vi "RIGOL_DS1202_continuous.vi"() -> ()   [LabVIEW 2021]
uses:
  <instrlib>/RIGOL DS1000 Series/Public/Data/Read (Single Waveform).vi
  <instrlib>/RIGOL DS1000 Series/RIGOL DS1000 Series.lvlib
panel:
  out "size(s)":i32
  in  "Channel (0: Channel 1)":u16(ring) items=["Channel 1", "Channel 2", "Channel 3", "Channel 4"]
  out "Waveform Data":waveform(dbl)(graph)={"t0"=timestamp(0 s since 1904-01-01), "dt"=2.0000000000000002e-07, "Y"=array[1202 elements]}
  in  "Stop":bool
  in  "Timeout (10000 ms)":u32=10000
  in  "VISA resource name":refnum<visa-resource-name>="USB0::0x1AB1::0x0517::DS1ZE244412916::INSTR"
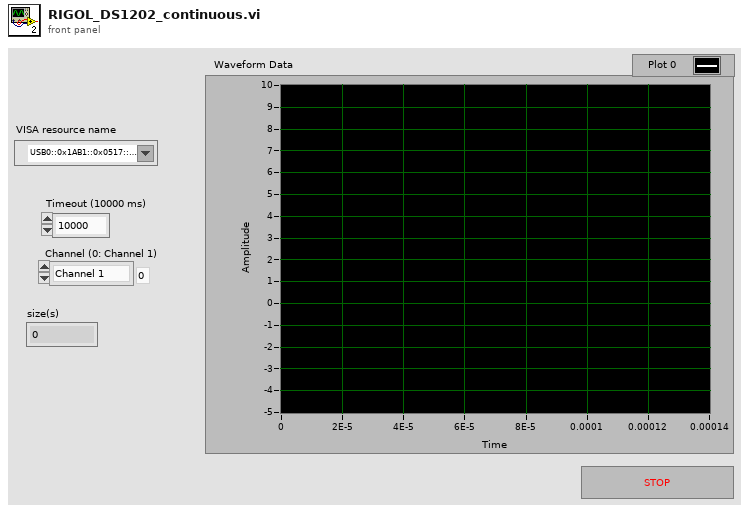
[diagram p1: front panel]
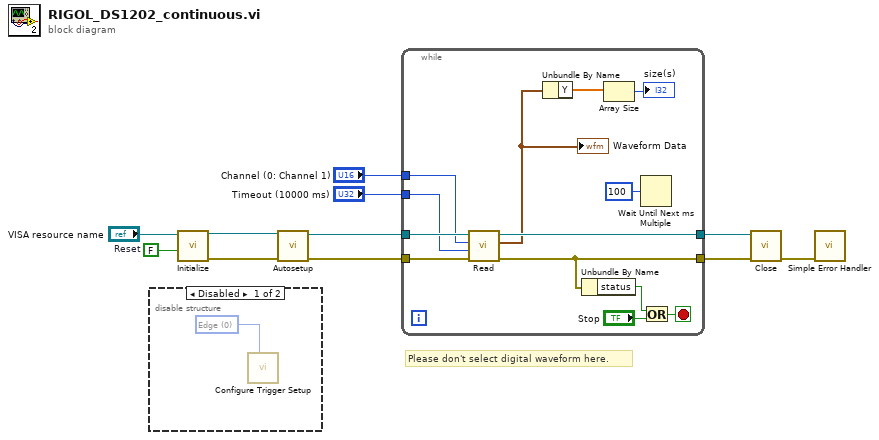
[diagram p0: block diagram]
diagram:
  w1 = FALSE  # Reset
  # "Please don't select digital waveform here."
  n1 = disable-structure shown="Disabled" {
    frame Disabled {
      w12 = u16 0 items=["Edge", "Pulse", "Video", "Pattern", "Duration"] ("Trigger Type (0: Edge)")
      n2 = call <instrlib>:"Configure Trigger Setup.vi"("Trigger Type (0: Edge)"=w12) -> ()  [unwired: 9 in, 2 out]
    }
    frame Enabled {
    }
  }
  n3 = call <instrlib>:"Initialize.vi"("Reset (True)"=w1, "VISA resource name"="VISA resource name") -> ("error out"=w6:errorcluster, "VISA resource name out"=w5:refnum<visa-resource-name>)  [unwired: 2 in, 6 out]
  n4 = call <instrlib>:"Autosetup.vi"("error in (no error)"=w6, "VISA resource name"=w5) -> ("error out"=w3:errorcluster, "VISA resource name out"=w4:refnum<visa-resource-name>)  [unwired: 8 out]
  n5 = while {
    tunnel: w4 -> [w25]
    tunnel: w3 -> [w24]
    tunnel: [w23] -> w10
    tunnel: [w20] -> w9
    tunnel: "Timeout (10000 ms)" -> [w16]
    tunnel: "Channel (0: Channel 1)" -> [w17]
    stop <- w21 stop-if-true
    n6 = call-poly <instrlib>:"Read.vi"("error in (no error)"=w24, "Timeout (10000 ms)"=w16, "Channel (0: Channel 1)"=w17, "VISA resource name"=w25) -> ("error out"=w20:errorcluster, "Waveform Data"=w15:waveform(dbl), "VISA resource name out"=w23:refnum<visa-resource-name>)  [unwired: 5 out]
    "Waveform Data" <- w15
    n7 = Unbundle By Name(w15) -> ("Y"=w14:dbl[])
    n8 = Unbundle By Name(w20) -> ("status"=w19:bool)
    n9 = Array Size(array=w14) -> (size(s)=→"size(s)":i32)
    n10 = Wait Until Next ms Multiple(millisecond multiple=u32 100) -> ()  [unwired: 1 out]
    n11 = Or(x=w19, y="Stop") -> (x .or. y?=w21:bool)
  }
  n12 = call <instrlib>:"Close.vi"("error in (no error)"=w9, "VISA resource name"=w10) -> ("error out"=w11:errorcluster)  [unwired: 9 out]
  n13 = call <vilib>:"Simple Error Handler.vi"("error in (no error)"=w11) -> ()  [unwired: 1 in, 8 out]
